vi "TransGenerate_v2.vi"() -> ()   [LabVIEW 2017]
uses:
  <vilib>/Analysis/NI_AALBase.lvlib
panel:
  in  "Cycles":dbl=1.0 format="%0.2f"
  in  "Noise":bool
  in  "A1":dbl step=100.0
  in  "tau1":dbl step=0.1
  out "Waveform Graph 4":dbl[][](graph)
  in  "Z":dbl
  in  "DNL\nAmplitude":dbl=1.0 format="%0.4f"
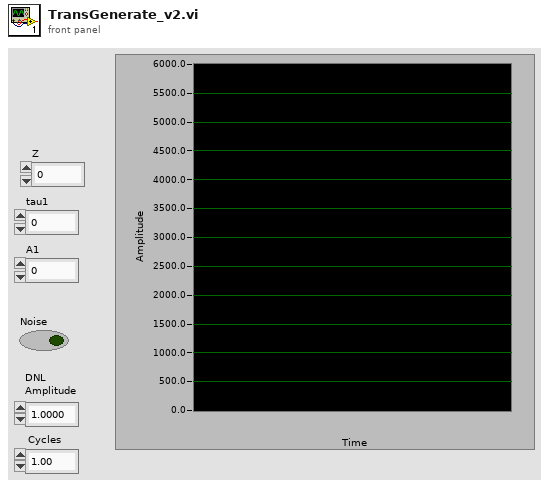
[diagram p1: front panel]
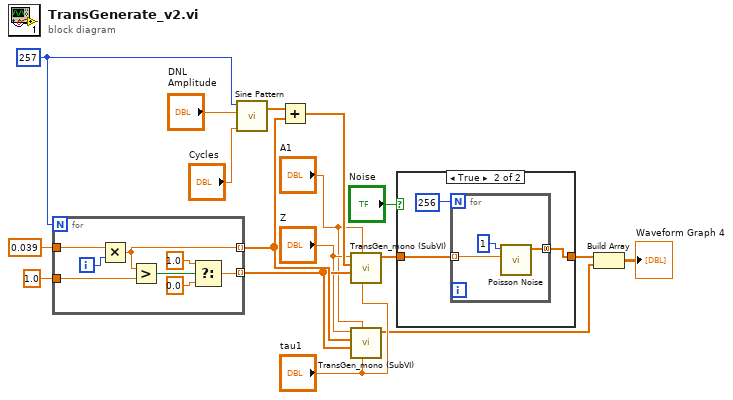
[diagram p0: block diagram]
diagram:
  w14 = 257
  n1 = for {
    N: w14 -> [_]
    tunnel: 0.039 ("x") -> [w24]
    tunnel: [w20] -> w8 mode=indexing
    tunnel: 1.0 ("y") -> [w23]
    tunnel: [w18] -> w7 mode=indexing
    i -> [w25]
    n2 = Multiply(x=w24, y=w25) -> (x*y=w20:dbl)
    n3 = Greater?(x=w20, y=w23) -> (0:w22:bool)
    n4 = Select(t=1.0, s=w22, f=0.0) -> (s? t:f=w18:dbl)
  }
  n5 = call <vilib>:"Sine Pattern.vi"("cycles"="Cycles", "amplitude"="DNL\nAmplitude", "samples"=w14) -> ("Sinusoidal Pattern"=w16:dbl[])  [unwired: 1 in, 1 out]
  n6 = Add(x=w16, y=w8) -> (x+y=w13:dbl[])
  n7 = call "TransGen_mono (SubVI).vi"("tau1"="tau1", "A1"="A1", "step"=w7, "time"=w13, "Z"="Z") -> ("intensity"=w11:dbl[])  [unwired: 6 in]
  n8 = call "TransGen_mono (SubVI).vi"("tau1"="tau1", "A1"="A1", "step"=w7, "time"=w8, "Z"="Z") -> ("intensity"=w2:dbl[])  [unwired: 6 in]
  n9 = case shown="True" "Noise" {
    tunnel: w11 -> [w26 w29]
    tunnel: [w26 w28] -> w3
    frame False {
    }
    frame True {
      n10 = for {
        N: 256 -> [_]
        tunnel: w29 -> [w32] mode=indexing
        tunnel: [w31] -> w28 mode=concatenating
        n11 = call <vilib>:"Poisson Noise.vi"("mean"=w32, "samples"=1) -> ("poisson noise"=w31:dbl[])  [unwired: 8 in, 1 out]
      }
    }
  }
  n12 = Build Array(w3, w2) -> (→"Waveform Graph 4":dbl[][])
